vi "Wheel States Segmentation.vi"(11 "calculated wheel states":T1[](array[typedef])) -> (0 "steering angles (rad)":dbl[](array[numeric]), 1 "caster wheel angles (rad)":dbl[](array[numeric]), 2 "caster angular velocities":dbl[](array[numeric]), 3 "forward angular velocities":dbl[](array[numeric]), 5 "wheel names":string[](array[string]))   [LabVIEW 2011]
uses:
  <vilib>/robotics/Steering/Wheel/Wheel State.ctl
  <vilib>/robotics/Steering/Wheel/NI_Robotics_Wheel.lvclass
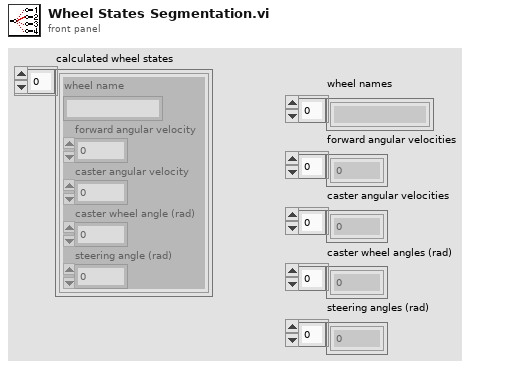
[diagram p1: front panel]
types:
  T1 = typedef "NI_Robotics_Wheel.lvclass/Wheel State.ctl" = cluster{"wheel name":string, "forward angular velocity":dbl, "caster angular velocity":dbl, "caster wheel angle (rad)":dbl, "steering angle (rad)":dbl}
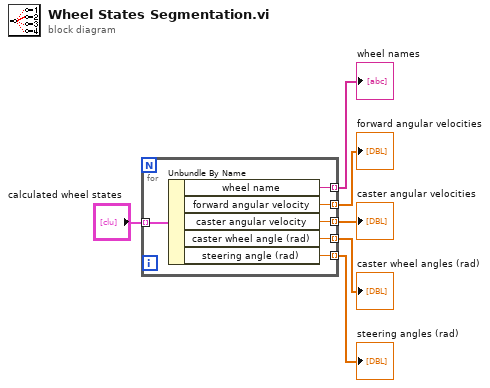
[diagram p0: block diagram]
diagram:
  n1 = for {
    tunnel: "calculated wheel states" -> [w12] mode=indexing
    tunnel: [w11] -> w5 mode=indexing
    tunnel: [w10] -> w4 mode=indexing
    tunnel: [w9] -> w1 mode=indexing
    tunnel: [w8] -> w2 mode=indexing
    tunnel: [w7] -> w3 mode=indexing
    n2 = Unbundle By Name(w12) -> ("wheel name"=w11:string, "forward angular velocity"=w10:dbl, "caster angular velocity"=w9:dbl, "caster wheel angle (rad)"=w8:dbl, "steering angle (rad)"=w7:dbl)
  }
  "caster wheel angles (rad)" <- w2
  "steering angles (rad)" <- w3
  "forward angular velocities" <- w4
  "wheel names" <- w5
  "caster angular velocities" <- w1
